vi "Get Column Info.vi"(8 "Error In":errorcluster, 11 "Table":string) -> (0 "Error Out":errorcluster, 2 "Column Information":T2(array[cluster]), 3 "Column Names":string[](array[string]))   [LabVIEW 2018, in "Database.lvlib"]
uses:
  Database.lvlib
  <vilib>/addons/database/Auxilliary.llb/DB Tools DataTypes.ctl
  Action.ctl
  <vilib>/addons/database/NI_Database_API.lvlib
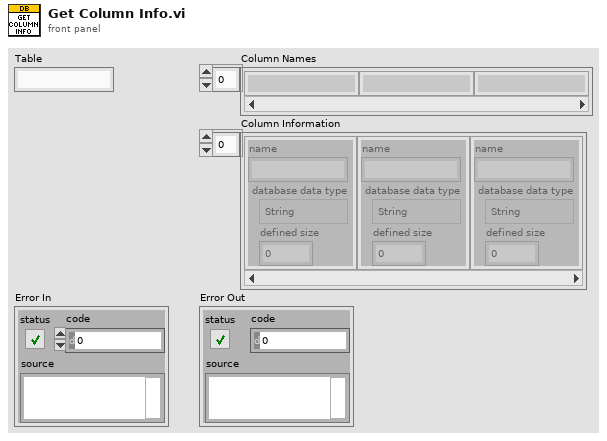
[diagram p1: front panel]
types:
  T1 = typedef "NI_Database_API.lvlib/DB Tools DataTypes.ctl" = enum16{"String", "Long (I32)", "Single (SGL)", "Double (DBL)", "Date/Time", "Binary"}
  T2 = cluster{"name":string, "database data type":T1, "defined size":i32}[]
  T3 = cluster{"column information":cluster{"name":string, "database data type":T1, "defined size":i32}[], "columns":string[]}
  T4 = typedef "Database.lvlib/Action.ctl" = enum16{"Init", "List Tables", "List Columns", "Query", "Close"}
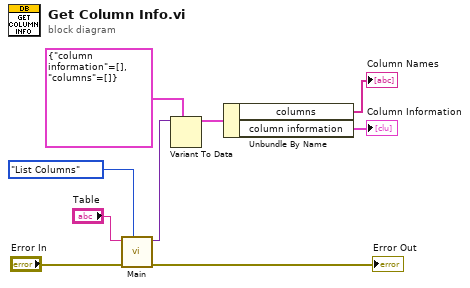
[diagram p0: block diagram]
diagram:
  n1 = call "Main.vi"("Action"=Action."List Columns", "Error In"="Error In", "Input"="Table") -> ("Error Out"=→"Error Out":errorcluster, "Output"=w5:variant)  [unwired: 7 in]
  n2 = Variant To Data(type=T3 {"column information"=[], "columns"=[]} ("cluster"), Variant=w5) -> (data=w7:T3)  [unwired: 1 in, 1 out]
  n3 = Unbundle By Name(w7) -> ("columns"=→"Column Names":string[], "column information"=→"Column Information":T2)
